vi "GraphLegendTlog.vi"(0 "XY Graph Ref":refnum<vi>, 5 "TracerCourbe":bool[](array[boolean]), 7 "Scan list":string[](array[string]), 11 "error in (no error)":errorcluster) -> (15 "error out":errorcluster)   [LabVIEW 2010]
doc: "Ce VI formatte la légende du graphique en fonction des paramètres d'acquisition choisis."
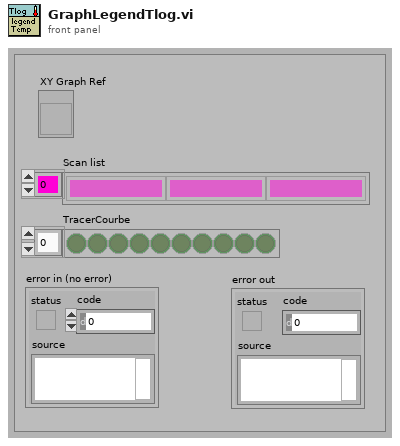
[diagram p1: front panel]
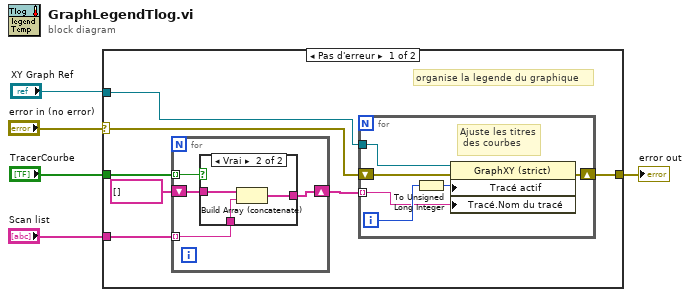
[diagram p0: block diagram]
diagram:
  n1 = case shown="Pas d'erreur" "error in (no error)" {
    selector: "error in (no error)" -> [w6 w27]
    tunnel: "XY Graph Ref" -> [w7 _]
    tunnel: "Scan list" -> [w10 _]
    tunnel: [w12 w27] -> w4
    tunnel: "TracerCourbe" -> [w11 _]
    frame No Error {
      # "organise la legende du graphique"
      n2 = for {
        tunnel: w11 -> [w14] mode=indexing
        tunnel: w10 -> [w16] mode=indexing
        shift-right: [w15] -> w9
        shift-left: string[] [] -> [w13]
        n3 = case shown="Vrai" w14 {
          tunnel: w16 -> [_ w20]
          tunnel: [w17 w19] -> w15
          tunnel: w13 -> [w17 w18]
          frame False {
          }
          frame True {
            n4 = Build Array (concatenate)(w18, w20) -> (w19:string[])
          }
        }
      }
      n5 = for {
        tunnel: w7 -> [w21]
        shift-right: [w26] -> w12
        shift-left: w6 -> [w23]
        tunnel: w9 -> [w22] mode=indexing
        i -> [w24]
        # "Ajuste les titres\n des courbes"
        n6 = To Unsigned Long Integer(number=w24) -> (unsigned 32bit integer=w25:u32)
        n7 = property class="GraphXY (strict)"(reference=w21, error in=w23, "Tracé actif"=w25, "Tracé.Nom du tracé"=w22) -> (error out=w26:errorcluster)  [unwired: 1 out]
      }
    }
    frame Error {
    }
  }
  "error out" <- w4
